vi "EncodeDecoded.vi"() -> ()   [LabVIEW 2019]
panel:
  in  "Private key":u8
  out "Decrypted string":string
  out "Encrypted string":string
  out "Encoded string":string
  in  "Input string":string
  out "Decoded string":string
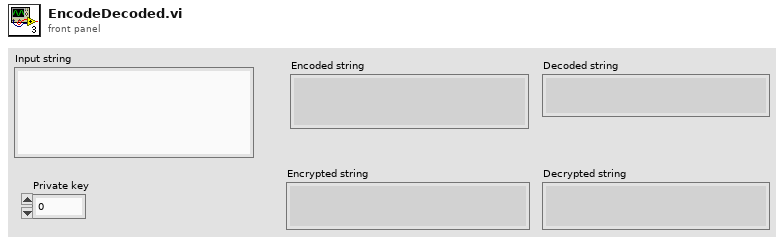
[diagram p1: front panel]
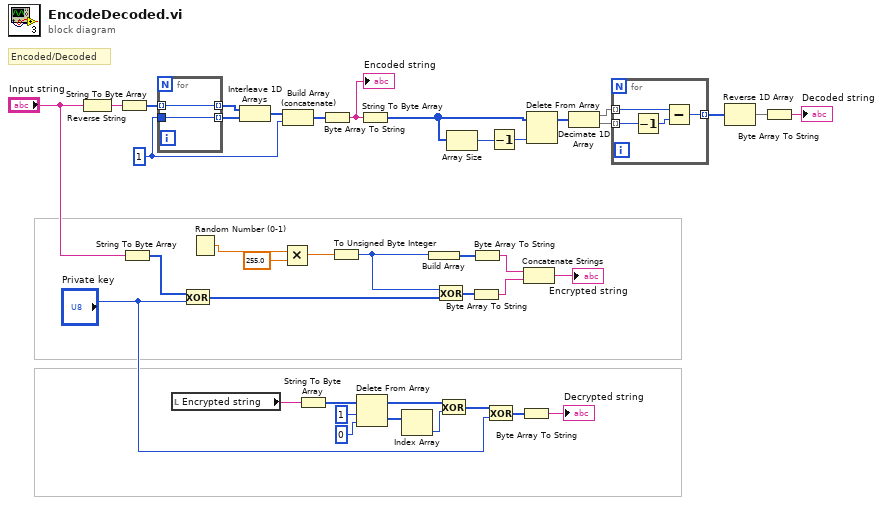
[diagram p0: block diagram]
diagram:
  w27 = u8 1
  # "Encoded/Decoded"
  n1 = Reverse String(1:"Input string") -> (0:w31:string)
  n2 = String To Byte Array(string=w31) -> (unsigned byte array=w24:u8[])
  n3 = String To Byte Array(string="Input string") -> (unsigned byte array=w3:u8[])
  n4 = for {
    tunnel: w24 -> [w42] mode=indexing
    tunnel: [w42] -> w30 mode=indexing
    tunnel: w27 -> [w41]
    tunnel: [w41] -> w29 mode=indexing
  }
  n5 = local read "Encrypted string"() -> (w1:string)
  n6 = Exclusive Or(1:"Private key", 2:w3) -> (0:w20:u8[])
  n7 = Random Number (0-1)() -> (number: 0 to 1=w23:dbl)
  n8 = Interleave 1D Arrays(w30, w29) -> (w28:u8[])
  n9 = Multiply(x=w23, y=255.0) -> (x*y=w21:dbl)
  n10 = Build Array (concatenate)(w28, w27) -> (w26:u8[])
  n11 = String To Byte Array(string=w1) -> (unsigned byte array=w2:u8[])
  n12 = Byte Array To String(unsigned byte array=w26) -> (string=w25:string)
  "Encoded string" <- w25
  n13 = To Unsigned Byte Integer(number=w21) -> (unsigned 8bit integer=w19:u8)
  n14 = Delete From Array(array=w2, length=1, index=0) -> (deleted portion=w10:u8[], array with subset deleted=w11:u8[])
  n15 = String To Byte Array(string=w25) -> (unsigned byte array=w36:u8[])
  n16 = Index Array(array=w10) -> (element=w9:u8)  [unwired: 1 in]
  n17 = Build Array(w19) -> (w18:u8[])
  n18 = Exclusive Or(1:w20, 2:w19) -> (0:w17:u8[])
  n19 = Exclusive Or(1:w9, 2:w11) -> (0:w8:u8[])
  n20 = Array Size(array=w36) -> (size(s)=w37:i32)
  n21 = Byte Array To String(unsigned byte array=w17) -> (string=w15:string)
  n22 = Byte Array To String(unsigned byte array=w18) -> (string=w16:string)
  n23 = Exclusive Or(1:"Private key", 2:w8) -> (0:w6:u8[])
  n24 = Decrement(x=w37) -> (x-1=w33:i32)
  n25 = Byte Array To String(unsigned byte array=w6) -> (string=→"Decrypted string":string)
  n26 = Concatenate Strings(w16, w15) -> (→"Encrypted string":string)
  n27 = Delete From Array(array=w36, index=w33) -> (array with subset deleted=w38:u8[])  [unwired: 1 in, 1 out]
  n28 = Decimate 1D Array(w38) -> (w39:u8[], w40:u8[])
  n29 = for {
    tunnel: w39 -> [w46] mode=indexing
    tunnel: [w45] -> w35 mode=indexing
    tunnel: w40 -> [w44] mode=indexing
    n30 = Decrement(x=w44) -> (x-1=w43:u8)
    n31 = Subtract(x=w46, y=w43) -> (x-y=w45:u8)
  }
  n32 = Reverse 1D Array(array=w35) -> (reversed array=w34:u8[])
  n33 = Byte Array To String(unsigned byte array=w34) -> (string=→"Decoded string":string)
